vi "Initialize Camera and CheckList.vi"(11 "ListBox in":refnum<vi>) -> ()   [LabVIEW 2019]
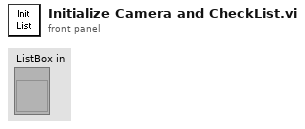
[diagram p1: front panel]
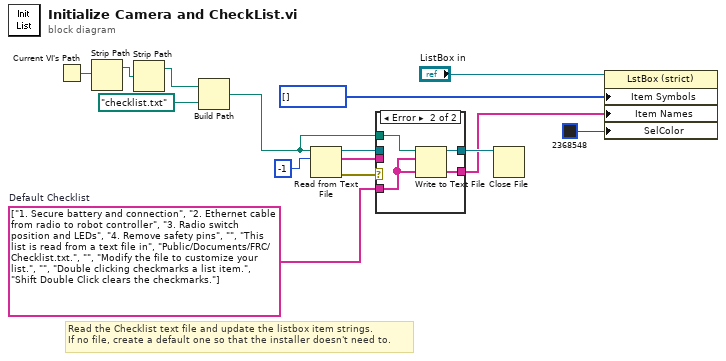
[diagram p0: block diagram]
diagram:
  w12 = string[] ["1. Secure battery and connection", "2. Ethernet cable from radio to robot controller", "3. Radio switch position and LEDs", "4. Remove safety pins", "", "This list is read from a text file in", "Public/Documents/FRC/Checklist.txt.", "", "Modify the file to customize your list.", "", "Double clicking checkmarks a list item.", "Shift Double Click clears the checkmarks."]  # Default Checklist
  # "Read the Checklist text file and update the listbox item strings.\nIf no file, create a default one so that the installer doesn't need to."
  n1 = Current VI's Path() -> (path=w5:path)
  n2 = Strip Path(path=w5) -> (stripped path=w4:path)  [unwired: 1 out]
  n3 = Strip Path(path=w4) -> (stripped path=w3:path)  [unwired: 1 out]
  n4 = Build Path(base path=w3, name or relative path=path "checklist.txt" ("XML File Path")) -> (appended path=w2:path)
  n5 = Read from Text File(file (use dialog)=w2, count=-1 ("timeout ms (25000)")) -> (refnum out=w14:refnum<file>, text=w11:string[], error out=w10:errorcluster)  [unwired: 2 in, 1 out]
  n6 = case shown="Error" w10 {
    tunnel: w11 -> [w17 _]
    tunnel: [w17 w19] -> w13
    tunnel: w12 -> [_ w19]
    tunnel: w2 -> [_ w20]
    tunnel: [w16 w18] -> w15
    tunnel: w14 -> [w16 _]
    frame No Error {
    }
    frame Error {
      n7 = Write to Text File(file (use dialog)=w20, text=w19) -> (refnum out=w18:refnum<file>)  [unwired: 2 in, 2 out]
    }
  }
  n8 = Close File(refnum=w15) -> ()  [unwired: 1 in, 2 out]
  n9 = property on="Property Node" class="LstBox (strict)"(reference="ListBox in", "Item Symbols"=i32[] [], "Item Names"=w13, "SelColor"=u32 2368548) -> ()  [unwired: 1 in, 2 out]
